vi "Generate Simulated Data.vi"(6 "Acquisition":refnum<queue>, 8 "error in (no error)":errorcluster, 10 "Longueur d'onde":dbl) -> (0 "error out":errorcluster, 2 "Data Out":variant[](array[variant]), 3 "Disconnected":bool=TRUE)   [LabVIEW 2018, in "Acquisition.lvlib"]
doc: "Generates sample waveforms according to the signal type in the HW Config input."
uses:
  Acquisition.lvlib
  <vilib>/Analysis/NI_AALBase.lvlib
  GlobalVariable/GlobalPowerByTime.vi
  GlobalVariable/Globalt0.vi
  support/Message Queue/Message Queue.lvlib
  <vilib>/gmath/NI_Gmath.lvlib
  GlobalVariable/GlobalSet0.vi
  <vilib>/Analysis/NI_AALPro.lvlib
  GlobalVariable/GlobalPosXbyTime.vi
  GlobalVariable/GlobalPosYbyTime.vi
  GlobalVariable/GlobalProfileByTime.vi
  GlobalVariable/GlobalTimeStep.vi
  GlobalVariable/GlobalTensionByTime.vi
  GlobalVariable/GlobalTemperatureByTime.vi
  <vilib>/numeric/Random Number (Range) I64.vi
  support/Message Queue/Enqueue Message (Single).vi
  <vilib>/gmath/interp.llb/Create Mesh Grid (2D) (x,y arrays).vi
  <vilib>/Analysis/2dsp.llb/2D Convolution (DBL).vi
  <vilib>/Analysis/baseanly.llb/Mean (DBL).vi
  <vilib>/DAQmx/create/channels.llb/DAQmx Create Channel (DO-Digital Output).vi
  <resource>/objmgr/daqmx.rc
  <vilib>/DAQmx/write.llb/DAQmx Write (Digital 1D Bool NChan 1Samp 1Line).vi
  <vilib>/DAQmx/read.llb/DAQmx Read (Analog 1D Wfm NChan NSamp).vi
  <vilib>/DAQmx/configure/timing.llb/DAQmx Timing (Sample Clock).vi
  <vilib>/DAQmx/create/channels.llb/DAQmx Create Channel (AI-Voltage-Basic).vi
  support/Message Queue/Message Cluster.ctl
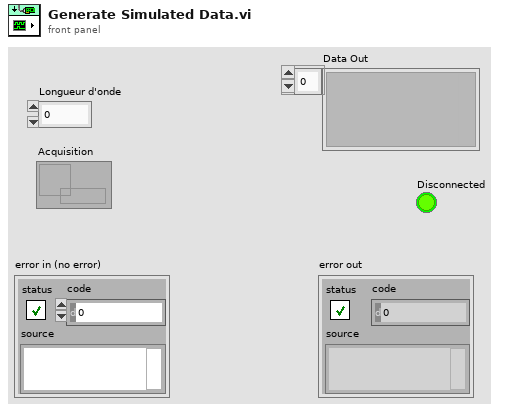
[diagram p1: front panel]
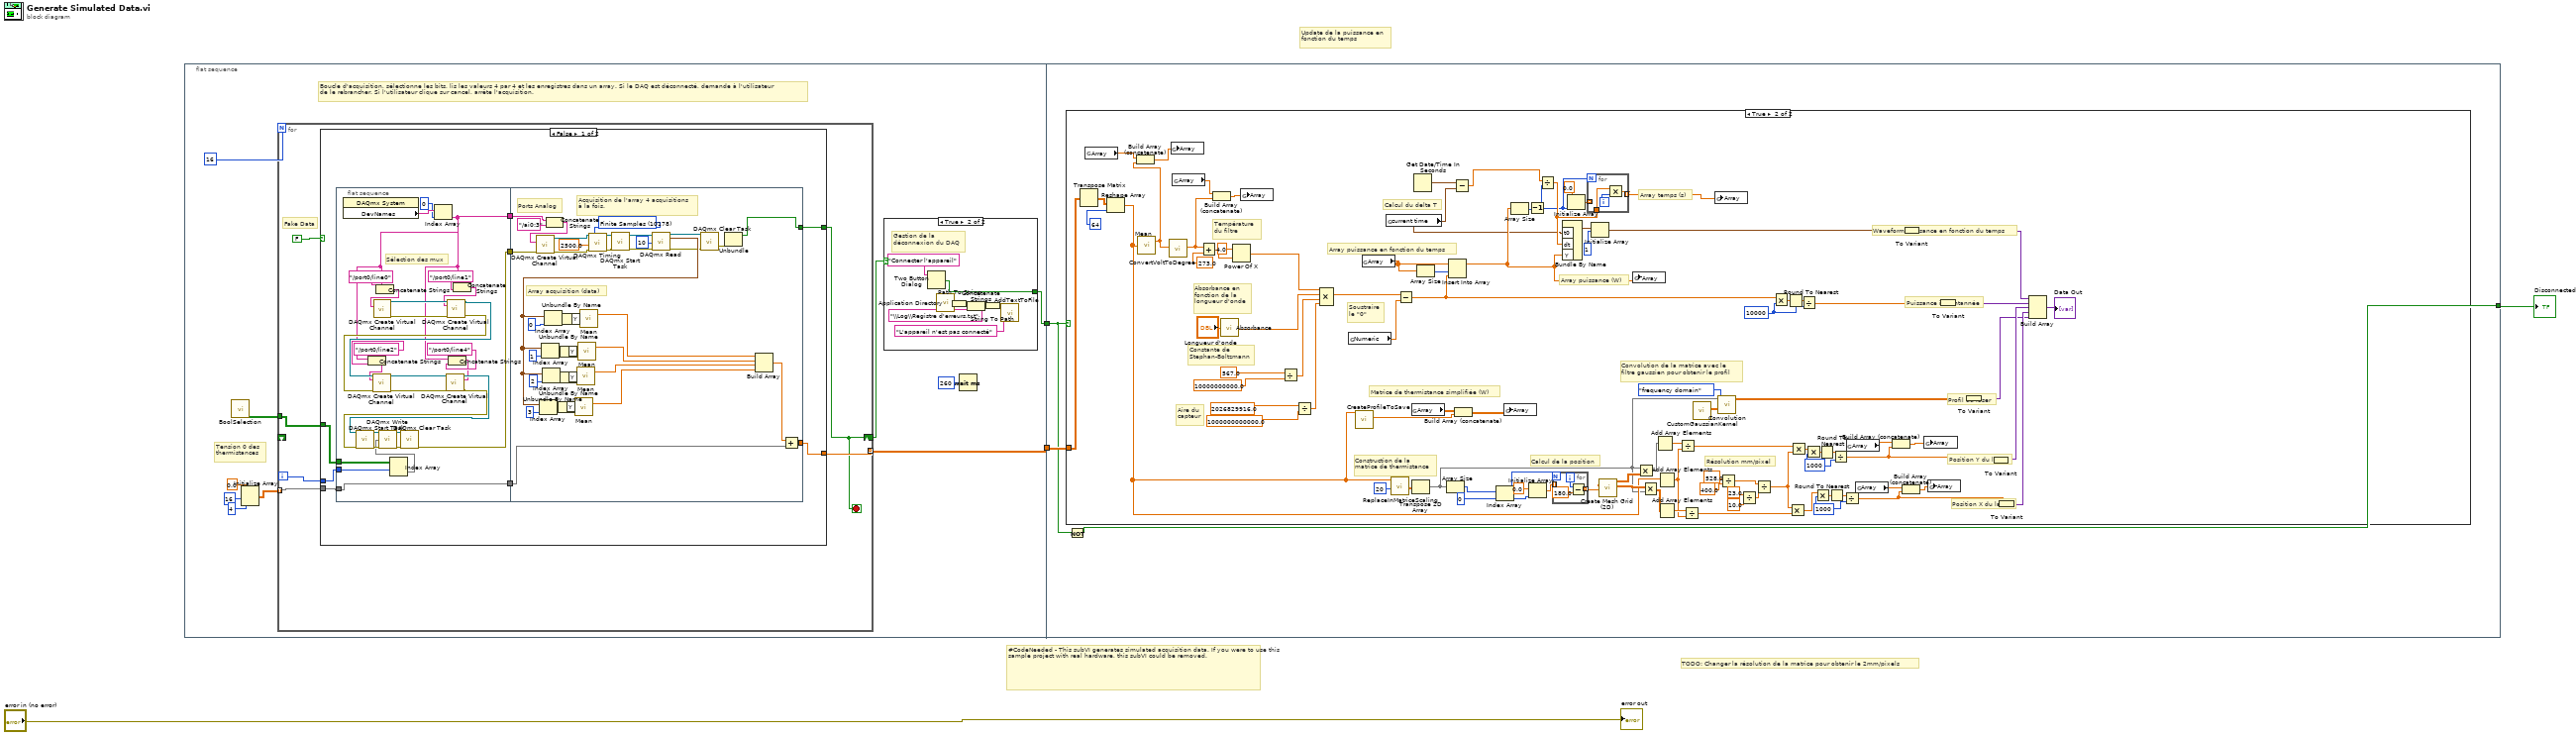
[diagram p0: block diagram]
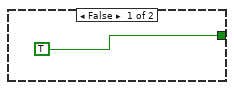
[diagram p2: hidden frame]
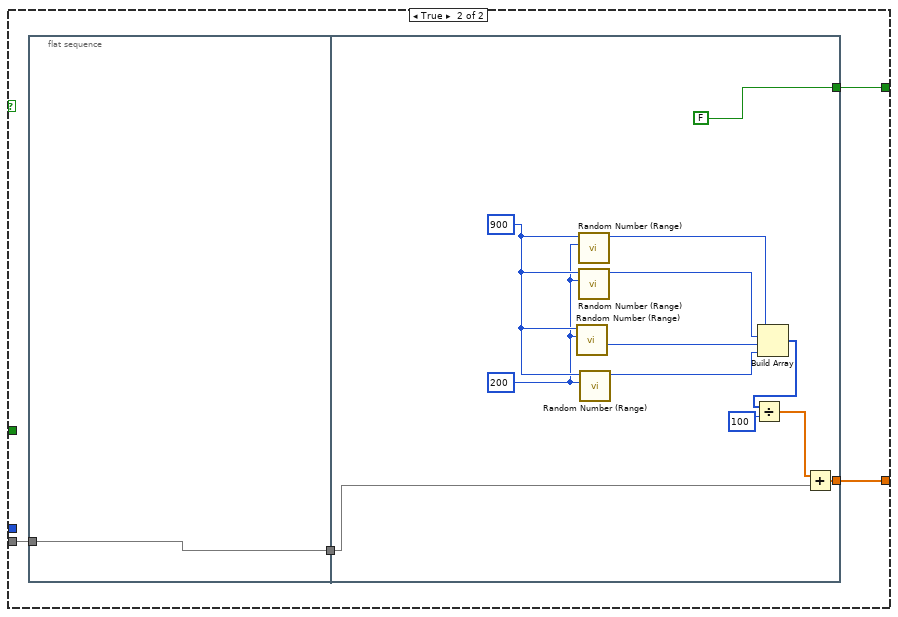
[diagram p3: hidden frame]
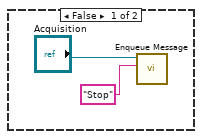
[diagram p4: hidden frame]
diagram:
  # "TODO: Changer la résolution de la matrice pour obtenir le 2mm/pixels"
  # "Update de la puissance en\nfonction du temps"
  # "#CodeNeeded - This subVI generates simulated acquisition data. If you were to use this sample project with real hardware, this subVI could be removed."
  n1 = flat-sequence {
    tunnel: [w12] -> w3
    tunnel: [w11] -> w2
    tunnel: w3 -> [w122]
    tunnel: w2 -> [w121]
    tunnel: [w120] -> w1
    frame #0 {
      # "Boucle d'acquisition, sélectionne les bits, lis les valeurs 4 par 4 et les enregistres dans un array. Si le DAQ est déconnecté, demande à l'utilisateur \nde le rebrancher. Si l'utilisateur clique sur cancel, arrête l'acquisition."
      # "Tension 0 des \nthermistances"
      n2 = call "BoolSelection.vi"() -> ("BoolSelection"=w13:bool[][])  [unwired: 11 in]
      n3 = Initialize Array(0.0 ("element"), 16 ("dimension size"), 4 ("dimension size")) -> (w7:dbl[][])
      n4 = for {
        N: 16 -> [_]
        tunnel: w13 -> [w26]
        tunnel: w7 -> [w29] mode=indexing
        tunnel: [w28] -> w12 mode=indexing
        shift-right: [w24] -> w6
        shift-left: _ -> [_]
        i -> [w25]
        stop <- w24 stop-if-true
        # "Fake Data"
        n5 = case shown="False" FALSE {
          tunnel: w29 -> [w32 w105]
          tunnel: [w30 w104] -> w28
          tunnel: [w31 w103] -> w24
          tunnel: w26 -> [w34 _]
          tunnel: w25 -> [w33 _]
          frame False {
            n6 = flat-sequence {
              tunnel: w33 -> [w51]
              tunnel: [w62] -> w37
              tunnel: w34 -> [w50]
              tunnel: [w38] -> w36
              tunnel: [w39] -> w35
              tunnel: w32 -> [w38]
              tunnel: w37 -> [w94]
              tunnel: w36 -> [w74]
              tunnel: [w76] -> w30
              tunnel: w35 -> [w71]
              tunnel: [w66] -> w31
              frame #0 {
                # "Sélection des mux"
                n7 = property class="DAQmx System"() -> ("DevNames"=w49:tag[])  [unwired: 2 in, 2 out]
                n8 = Index Array(array=w50, index (row)=w51) -> (element=w63:bool[])  [unwired: 1 in]
                n9 = Index Array(array=w49, index=0) -> (element=w39:tag)
                n10 = Concatenate Strings(w39, "/port0/line2" ("string")) -> (w42:string)
                n11 = Concatenate Strings(w39, "/port0/line0" ("string")) -> (w47:string)
                n12 = call-poly <vilib>:"DAQmx Create Virtual Channel.vi"("lines"=w47) -> ("task out"=w58:refnum<k21>, "error out"=w59:errorcluster)  [unwired: 13 in]
                n13 = Concatenate Strings(w39, "/port0/line4" ("string")) -> (w40:string)
                n14 = Concatenate Strings(w39, "/port0/line1" ("string")) -> (w44:string)
                n15 = call-poly <vilib>:"DAQmx Create Virtual Channel.vi"("task in"=w58, "lines"=w44, "error in"=w59) -> ("task out"=w57:refnum<k21>, "error out"=w56:errorcluster)  [unwired: 11 in]
                n16 = call-poly <vilib>:"DAQmx Create Virtual Channel.vi"("task in"=w57, "lines"=w42, "error in"=w56) -> ("task out"=w54:refnum<k21>, "error out"=w55:errorcluster)  [unwired: 11 in]
                n17 = call-poly <vilib>:"DAQmx Create Virtual Channel.vi"("task in"=w54, "lines"=w40, "error in"=w55) -> ("task out"=w53:refnum<k21>, "error out"=w52:errorcluster)  [unwired: 11 in]
                n18 = call <vilib>:"DAQmx Start Task.vi"("task/channels in"=w53, "error in"=w52) -> ("task out"=w64:refnum<k21>, "error out"=w65:errorcluster)  [unwired: 12 in]
                n19 = call-poly <vilib>:"DAQmx Write.vi"("task/channels in"=w64, "data"=w63, "error in"=w65) -> ("task out"=w61:refnum<k21>, "error out"=w60:errorcluster)  [unwired: 10 in, 1 out]
                n20 = call <vilib>:"DAQmx Clear Task.vi"("task in"=w61, "error in"=w60) -> ("error out"=w62:errorcluster)  [unwired: 13 in]
              }
              frame #1 {
                w96 = 10178 items=["Finite Samples"=10178, "Continuous Samples"=10123, "Hardware Timed Single Point"=12522] ("sample mode")
                # "Ports Analog"
                # "Array acquisition (data)"
                # "Acquisition de l'array 4 acquisitions\nà la fois."
                n21 = Concatenate Strings(w71, "/ai0:3" ("string")) -> (w72:string)
                n22 = call-poly <vilib>:"DAQmx Create Virtual Channel.vi"("physical channels"=w72, "error in"=w94) -> ("task out"=w101:refnum<k21>, "error out"=w100:errorcluster)  [unwired: 12 in]
                n23 = call-poly <vilib>:"DAQmx Timing.vi"("task/channels in"=w101, "sample mode"=w96, "rate"=2500.0, "error in"=w100) -> ("task out"=w97:refnum<k21>, "error out"=w98:errorcluster)  [unwired: 10 in]
                n24 = call <vilib>:"DAQmx Start Task.vi"("task/channels in"=w97, "error in"=w98) -> ("task out"=w99:refnum<k21>, "error out"=w102:errorcluster)  [unwired: 12 in]
                n25 = call-poly <vilib>:"DAQmx Read.vi"("task/channels in"=w99, "number of samples per channel"=10, "error in"=w102) -> ("task out"=w78:refnum<k21>, "data"=w87:waveform(dbl)[], "error out"=w77:errorcluster)  [unwired: 10 in]
                n26 = Index Array(array=w87, index=3) -> (element=w83:waveform(dbl))
                n27 = Index Array(array=w87, index=1) -> (element=w85:waveform(dbl))
                n28 = Index Array(array=w87, index=2) -> (element=w84:waveform(dbl))
                n29 = Index Array(array=w87, index=0) -> (element=w86:waveform(dbl))
                n30 = Unbundle By Name(w83) -> ("Y"=w79:dbl[])
                n31 = Unbundle By Name(w85) -> ("Y"=w81:dbl[])
                n32 = Unbundle By Name(w84) -> ("Y"=w80:dbl[])
                n33 = Unbundle By Name(w86) -> ("Y"=w82:dbl[])
                n34 = call-poly <vilib>:"Mean.vi"("X"=w79) -> ("mean"=w67:dbl)  [unwired: 1 out]
                n35 = call-poly <vilib>:"Mean.vi"("X"=w80) -> ("mean"=w68:dbl)  [unwired: 1 out]
                n36 = call-poly <vilib>:"Mean.vi"("X"=w81) -> ("mean"=w69:dbl)  [unwired: 1 out]
                n37 = call-poly <vilib>:"Mean.vi"("X"=w82) -> ("mean"=w70:dbl)  [unwired: 1 out]
                n38 = call <vilib>:"DAQmx Clear Task.vi"("task in"=w78, "error in"=w77) -> ("error out"=w92:errorcluster)  [unwired: 13 in]
                n39 = Unbundle(w92) -> ("status"=w66:bool)  [unwired: 2 out]
                n40 = Build Array(w70, w69, w68, w67) -> (w75:dbl[])
                n41 = Add(x=w75, y=w74) -> (x+y=w76:dbl[])
              }
            }
          }
          frame True {
            n42 = flat-sequence {
              tunnel: [w107] -> w106
              tunnel: w105 -> [w107]
              tunnel: w106 -> [w114]
              tunnel: [w115] -> w104
              tunnel: [FALSE] -> w103
              frame #0 {
              }
              frame #1 {
                w111 = 200
                w112 = 900
                n43 = call-poly <vilib>:"Random Number (Range).vi"("lower bound (-100)"=w111, "upper bound (100)"=w112) -> ("number"=w116:i64)  [unwired: 9 in]
                n44 = call-poly <vilib>:"Random Number (Range).vi"("lower bound (-100)"=w111, "upper bound (100)"=w112) -> ("number"=w118:i64)  [unwired: 9 in]
                n45 = call-poly <vilib>:"Random Number (Range).vi"("lower bound (-100)"=w111, "upper bound (100)"=w112) -> ("number"=w119:i64)  [unwired: 9 in]
                n46 = call-poly <vilib>:"Random Number (Range).vi"("lower bound (-100)"=w111, "upper bound (100)"=w112) -> ("number"=w117:i64)  [unwired: 9 in]
                n47 = Build Array(w118, w119, w116, w117) -> (w109:i64[])
                n48 = Divide(x=w109, y=100) -> (x/y=w108:dbl[])
                n49 = Add(x=w108, y=w114) -> (x+y=w115:dbl[])
              }
            }
          }
        }
      }
      n50 = case shown="True" w6 {
        tunnel: [TRUE w23] -> w11
        frame False {
        }
        frame True {
          # "Gestion de la \ndéconnexion du DAQ"
          n51 = Two Button Dialog(message="Connecter l'appareil") -> (T button?=w23:bool)  [unwired: 2 in]
          n52 = call <vilib>:"Application Directory.vi"() -> ("Application Directory"=w20:path)
          n53 = Path To String(path=w20) -> (string=w21:string)
          n54 = Concatenate Strings(w21, "\\Log\\Registre d'erreurs.txt") -> (w22:string)
          n55 = String To Path(string=w22) -> (path=w18:path)
          n56 = call "AddTextToFile.vi"("Ajouter du texte"="L'appareil n'est pas connecté", "Fichier"=w18) -> ()  [unwired: 10 in]
        }
      }
      n57 = Wait (ms)(milliseconds to wait=u32 260) -> ()  [unwired: 1 out]
    }
    frame #1 {
      n58 = case shown="True" w121 {
        tunnel: w122 -> [_ w158]
        frame False {
          n59 = call-poly "Enqueue Message.vi"("Message"="Stop", "Message Queue"="Acquisition") -> ()  [unwired: 8 in, 2 out]
        }
        frame True {
          w169 = 1000
          w173 = 1000
          w179 = 10000
          # "Résolution mm/pixel"
          # "Calcul du delta T"
          # "Matrice de thermistance simplifiée (W)"
          # "Soustraire\nle \"0\""
          # "Constante de \nStephan-Boltzmann"
          # "Absorbance en\nfonction de la \nlongueur d'onde"
          # "Température \ndu filtre"
          # "Aire du\ncapteur"
          # "Calcul de la position"
          # "Construction de la \nmatrice de thermistance"
          # "Position X du laser"
          # "Position Y du laser"
          # "Profil du laser"
          # "Puissance instantannée"
          # "Waveform puissance en fonction du temps"
          # "Array puissance (W)"
          # "Array temps (s)"
          # "Convolution de la matrice avec le \nfiltre gaussien pour obtenir le profil"
          # "Array puissance en fonction du temps"
          n60 = Transpose Matrix(1:w158) -> (0:w159:dbl[][])
          n61 = global read "GlobalTensionByTime.vi" "Array"() -> (w137:dbl[])
          n62 = Reshape Array(w159, 64 ("dimension size")) -> (w154:dbl[])
          n63 = call-poly <vilib>:"Mean.vi"("X"=w154) -> ("mean"=w135:dbl)  [unwired: 1 out]
          n64 = Build Array (concatenate)(w137, w135) -> (w136:dbl[])
          n65 = call "ConvertVoltToDegree.vi"("Tension"=w135) -> ("Température"=w132:dbl)  [unwired: 10 in]
          n66 = global write "GlobalTensionByTime.vi" "Array"(w136) -> ()
          n67 = global read "GlobalTemperatureByTime.vi" "Array"() -> (w133:dbl[])
          n68 = Add(x=w132, y=273.0) -> (x+y=w207:dbl)
          n69 = Build Array (concatenate)(w133, w132) -> (w134:dbl[])
          n70 = call "Absorbance.vi"("Longueur d'onde"="Longueur d'onde") -> ("absorbance"=w162:dbl)  [unwired: 10 in]
          n71 = Power Of X(1:w207, 2:4.0 ("y")) -> (0:w161:dbl)
          n72 = global write "GlobalTemperatureByTime.vi" "Array"(w134) -> ()
          n73 = Divide(x=567.0, y=10000000000.0) -> (x/y=w163:dbl)
          n74 = Divide(x=2026829916.0, y=1000000000000.0) -> (x/y=w164:dbl)
          n75 = Compound Arithmetic op=MULTIPLY(w161, w162, w163, w164) -> (w157:dbl)
          n76 = global read "GlobalSet0.vi" "Numeric"() -> (w156:dbl)
          n77 = call "CreateProfileToSave.vi"("Input Array"=w154) -> ("Ouput array"=w144:dbl[])  [unwired: 10 in]
          n78 = global read "GlobalPowerByTime.vi" "Array"() -> (w219:dbl[])
          n79 = global read "Globalt0.vi" "current time"() -> (w139:timestamp)
          n80 = call "ReplaceInMatriceScaling.vi"("Input Scaling"=20, "Input Array"=w154) -> ("Output Array"=w214:dbl[][])  [unwired: 9 in]
          n81 = Subtract(x=w157, y=w156) -> (x-y=w155:dbl)
          n82 = global read "GlobalProfileByTime.vi" "Array"() -> (w143:dbl[][])
          n83 = Transpose 2D Array(2D array=w214) -> (transposed array=w126:dbl[][])
          n84 = Get Date/Time In Seconds() -> (seconds since 1Jan1904=w140:timestamp)
          n85 = Array Size(array=w219) -> (size(s)=w218:i32)
          n86 = Array Size(array=w126) -> (size(s)=w201:i32[])
          n87 = Insert Into Array(array=w219, index=w218, new element=w155) -> (w153:dbl[])
          n88 = Subtract(x=w140, y=w139) -> (x-y=w138:dbl)
          n89 = Build Array (concatenate)(w143, w144) -> (w145:dbl[][])
          n90 = Index Array(array=w201, index=0) -> (element=w196:i32)
          n91 = global write "GlobalProfileByTime.vi" "Array"(w145) -> ()
          n92 = Array Size(array=w153) -> (size(s)=w142:i32)
          n93 = Decrement(x=w142) -> (x-1=w141:i32)
          n94 = Initialize Array(0.0 ("element"), w196) -> (w198:dbl[])
          n95 = Divide(x=w138, y=w141) -> (x/y=w212:dbl)
          n96 = for {
            N: w196 -> [_]
            tunnel: w198 -> [_] mode=indexing
            tunnel: [w220] -> w193 mode=indexing
            i -> [w221]
            n97 = Subtract(x=w221, y=180.0) -> (x-y=w220:dbl)
          }
          n98 = Bundle By Name("t0"=w139, "dt"=w212, "Y"=w153) -> (w216:waveform(dbl))  [unwired: 1 in]
          n99 = Initialize Array(0.0 ("element"), w141) -> (w210:dbl[])
          n100 = for {
            N: w141 -> [_]
            tunnel: w212 -> [w224]
            tunnel: w210 -> [_] mode=indexing
            tunnel: [w223] -> w152 mode=indexing
            i -> [w225]
            n101 = Multiply(x=w224, y=w225) -> (x*y=w223:dbl)
          }
          n102 = Initialize Array(w216, 1) -> (w183:waveform(dbl)[])
          n103 = call-poly <vilib>:"Create Mesh Grid (2D).vi"("y domain"=w193, "x domain"=w193) -> ("Y"=w192:dbl[][], "X"=w197:dbl[][])  [unwired: 7 in, 1 out]
          n104 = global write "GlobalPowerByTime.vi" "Array"(w153) -> ()
          n105 = Multiply(x=w126, y=w197) -> (x*y=w195:dbl[][])
          n106 = Multiply(x=w192, y=w126) -> (x*y=w191:dbl[][])
          n107 = Add Array Elements(numeric array=w195) -> (sum=w194:dbl)
          n108 = Add Array Elements(numeric array=w154) -> (sum=w189:dbl)
          n109 = Add Array Elements(numeric array=w191) -> (sum=w190:dbl)
          n110 = Divide(x=w194, y=w189) -> (x/y=w187:dbl)
          n111 = Divide(x=w190, y=w189) -> (x/y=w188:dbl)
          n112 = call "CustomGaussianKernel.vi"() -> ("array"=w209:dbl[][])  [unwired: 11 in]
          n113 = global write "GlobalTimeStep.vi" "Array"(w152) -> ()
          n114 = call-poly <vilib>:"Convolution.vi"("algorithm"=enum32{"direct", "frequency domain"}."frequency domain", "Y"=w209, "X"=w126) -> ("X * Y"=w125:dbl[][])  [unwired: 7 in, 1 out]
          n115 = Divide(x=528.0, y=400.0) -> (x/y=w129:dbl)
          n116 = Divide(x=23.0 ("y"), y=10.0) -> (x/y=w128:dbl)
          n117 = Divide(x=w129, y=w128) -> (x/y=w127:dbl)
          n118 = Multiply(x=w155, y=w179) -> (x*y=w180:dbl)
          n119 = Round To Nearest(number=w180) -> (nearest integer value=w178:dbl)
          n120 = Multiply(x=w127, y=w188) -> (x*y=w166:dbl)
          n121 = Multiply(x=w187, y=w127) -> (x*y=w170:dbl)
          n122 = Divide(x=w178, y=w179) -> (x/y=w174:dbl)
          n123 = Multiply(x=w170, y=w173) -> (x*y=w172:dbl)
          n124 = Multiply(x=w166, y=w169) -> (x*y=w168:dbl)
          n125 = Round To Nearest(number=w172) -> (nearest integer value=w171:dbl)
          n126 = Round To Nearest(number=w168) -> (nearest integer value=w167:dbl)
          n127 = Divide(x=w171, y=w173) -> (x/y=w146:dbl)
          n128 = Divide(x=w167, y=w169) -> (x/y=w150:dbl)
          n129 = global read "GlobalPosXbyTime.vi" "Array"() -> (w147:dbl[])
          n130 = global read "GlobalPosYbyTime.vi" "Array"() -> (w151:dbl[])
          n131 = Build Array (concatenate)(w147, w146) -> (w148:dbl[])
          n132 = Build Array (concatenate)(w151, w150) -> (w149:dbl[])
          n133 = To Variant(anything=w183) -> (Variant=w182:variant)
          n134 = global write "GlobalPosXbyTime.vi" "Array"(w148) -> ()
          n135 = global write "GlobalPosYbyTime.vi" "Array"(w149) -> ()
          n136 = To Variant(anything=w174) -> (Variant=w175:variant)
          n137 = To Variant(anything=w125) -> (Variant=w165:variant)
          n138 = To Variant(anything=w146) -> (Variant=w176:variant)
          n139 = To Variant(anything=w150) -> (Variant=w177:variant)
          n140 = Build Array(w182, w175, w176, w177, w165) -> (→"Data Out":variant[])
        }
      }
      n141 = Not(x=w121) -> (.not. x?=w120:bool)
    }
  }
  "error out" <- "error in (no error)"
  "Disconnected" <- w1
